vi "setNumberOfWheels.vi"(8 "error in (no error)":errorcluster, 10 "numberOfWheels":dbl, 11 "bus in":refnum<class "bus.lvclass">) -> (0 "error out":errorcluster, 3 "bus out":refnum<class "bus.lvclass">)   [LabVIEW 2011, in "bus.lvclass"]
uses:
  bus.lvclass
  genericVehicle.lvclass
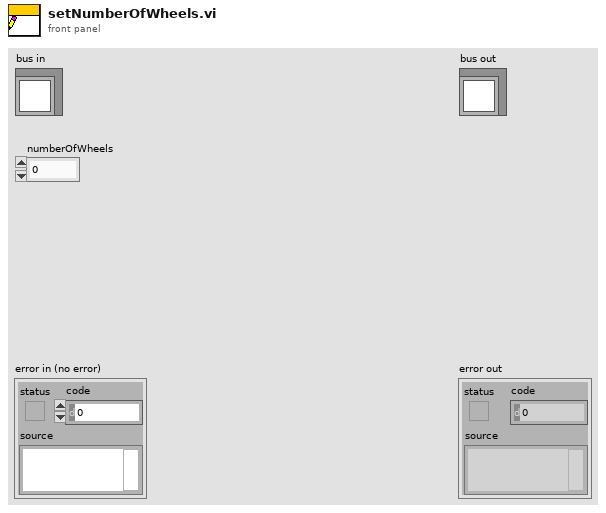
[diagram p1: front panel]
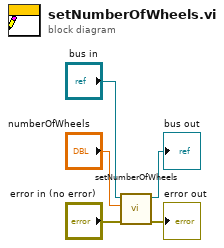
[diagram p0: block diagram]
diagram:
  n1 = call-parent "setNumberOfWheels.vi"("error in (no error)"="error in (no error)", "numberOfWheels"="numberOfWheels", "genericVehicle in"="bus in") -> ("error out"=→"error out":errorcluster, "genericVehicle out"=→"bus out":refnum<class "bus.lvclass">)  [unwired: 7 in]
